vi "QueryServer_Stop.vi"(0 "Server Info":T2, 2 "Event Registration Refnum":refnum<event-registration>, 3 "error in (no error)":errorcluster) -> (10 "error out":errorcluster)   [LabVIEW 2019, in "labview-grpc-query-server.lvlib"]
uses:
  labview-grpc-query-server.lvlib
  QueryServer_InvokeEventData.ctl
  VIs/grpcId.ctl
  VIs/gprc-support.lvlib
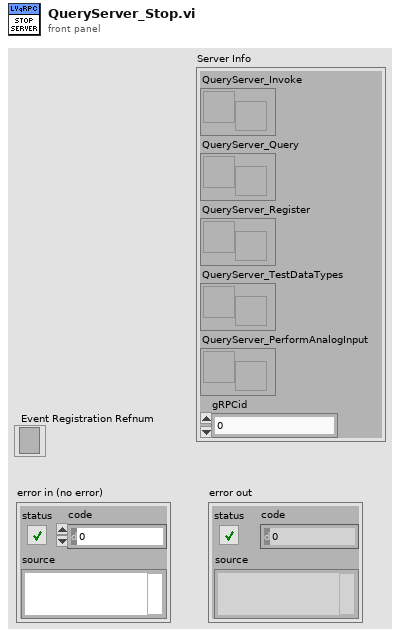
[diagram p1: front panel]
types:
  T1 = typedef "gprc-support.lvlib/grpcId.ctl" = u64
  T2 = cluster{"QueryServer_Invoke":refnum<user-event>, "QueryServer_Query":refnum<user-event>, "QueryServer_Register":refnum<user-event>, "QueryServer_TestDataTypes":refnum<user-event>, "QueryServer_PerformAnalogInput":refnum<user-event>, "gRPCid":T1}
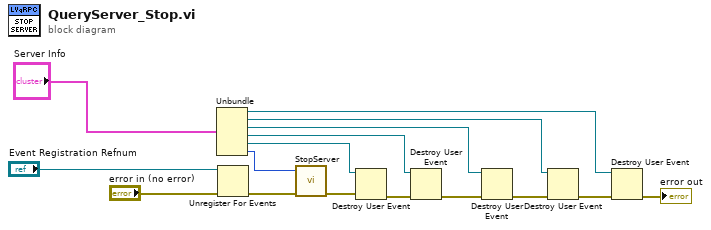
[diagram p0: block diagram]
diagram:
  n1 = Unbundle("Server Info") -> ("QueryServer_Invoke"=w10:refnum<user-event>, "QueryServer_Query"=w11:refnum<user-event>, "QueryServer_Register"=w12:refnum<user-event>, "QueryServer_TestDataTypes"=w8:refnum<user-event>, "QueryServer_PerformAnalogInput"=w2:refnum<user-event>, "gRPCid"=w5:T1)
  n2 = Unregister For Events(event registration refnum="Event Registration Refnum", error in="error in (no error)") -> (error out=w7:errorcluster)
  n3 = call "StopServer.vi"("error in (no error)"=w7, "Server Id"=w5) -> ("error out"=w4:errorcluster)  [unwired: 9 in]
  n4 = Destroy User Event(user event=w2, error in=w4) -> (error out=w3:errorcluster)
  n5 = Destroy User Event(user event=w8, error in=w3) -> (error out=w9:errorcluster)
  n6 = Destroy User Event(user event=w12, error in=w9) -> (error out=w15:errorcluster)
  n7 = Destroy User Event(user event=w11, error in=w15) -> (error out=w14:errorcluster)
  n8 = Destroy User Event(user event=w10, error in=w14) -> (error out=→"error out":errorcluster)
